vi "Read Measurement.vi"(8 "error in (no error)":errorcluster, 10 "Timeout (10000 ms)":u32=10000, 11 "VISA resource name":refnum<visa-resource-name>) -> (0 "error out":errorcluster, 2 "Measurement":dbl, 3 "VISA resource name out":refnum<visa-resource-name>)   [LabVIEW 2018, in "Agilent U2000 Series.lvlib"]
doc: "Performs a single, new measurement and outputs the result.\n\nNote: \nThe type of measurement returned is determined by calling the Configure Measurement VI."
uses:
  Agilent U2000 Series.lvlib
  Low Level/Initiate (Immediate).vi
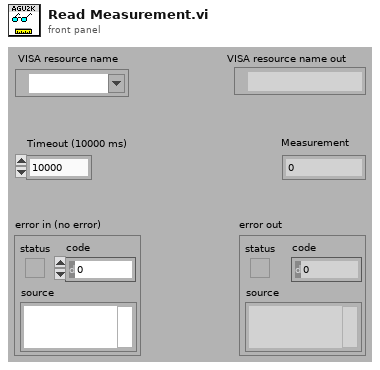
[diagram p1: front panel]
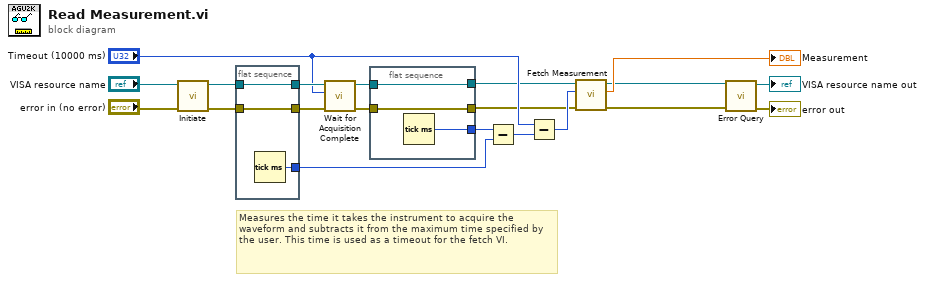
[diagram p0: block diagram]
diagram:
  # "Measures the time it takes the instrument to acquire the waveform and subtracts it from the maximum time specified by the user. This time is used as a timeout for the fetch VI."
  n1 = call-poly "Initiate.vi"("error in (no error)"="error in (no error)", "VISA resource name"="VISA resource name") -> ("error out"=w12:errorcluster, "VISA resource name out"=w13:refnum<visa-resource-name>)  [unwired: 8 in]
  n2 = flat-sequence {
    tunnel: [w23] -> w9
    tunnel: w13 -> [w23]
    tunnel: [w22] -> w10
    tunnel: w12 -> [w22]
    tunnel: [w21] -> w11
    frame #0 {
      n3 = Tick Count (ms)() -> (millisecond timer value=w21:u32)
    }
  }
  n4 = call "Wait for Acquisition Complete.vi"("error in (no error)"=w10, "Maximum Time (10000 ms)"="Timeout (10000 ms)", "VISA resource name"=w9) -> ("error out"=w6:errorcluster, "VISA resource name out"=w7:refnum<visa-resource-name>)  [unwired: 7 out]
  n5 = flat-sequence {
    tunnel: [w26] -> w4
    tunnel: w7 -> [w26]
    tunnel: [w25] -> w3
    tunnel: w6 -> [w25]
    tunnel: [w24] -> w5
    frame #0 {
      n6 = Tick Count (ms)() -> (millisecond timer value=w24:u32)
    }
  }
  n7 = Subtract(x=w5, y=w11) -> (x-y=w16:u32)
  n8 = Subtract(x="Timeout (10000 ms)", y=w16) -> (x-y=w14:u32)
  n9 = call "Fetch Measurement.vi"("error in (no error)"=w3, "Timeout (10000 ms)"=w14, "VISA resource name"=w4) -> ("error out"=w1:errorcluster, "Measurement"=→"Measurement":dbl, "VISA resource name out"=w2:refnum<visa-resource-name>)  [unwired: 6 out]
  n10 = call "Error Query.vi"("error in (no error)"=w1, "VISA resource name"=w2) -> ("error out"=→"error out":errorcluster, "VISA resource name out"=→"VISA resource name out":refnum<visa-resource-name>)  [unwired: 8 out]
